vi "CC命令发送.vi"(8 "error in (no error)":errorcluster caption="错误输入（无错误）", 11 "MainPage 输入":refnum<class "MainPage.lvclass">) -> (0 "error out":errorcluster caption="错误输出", 3 "MainPage 输出":refnum<class "MainPage.lvclass">)   [LabVIEW 2019, in "MainPage.lvlib" / "MainPage.lvclass"]
uses:
  MainPage.lvclass
  MainPage.lvclass/MainPage.ctl
panel:
  # "简略版本，后续修改"
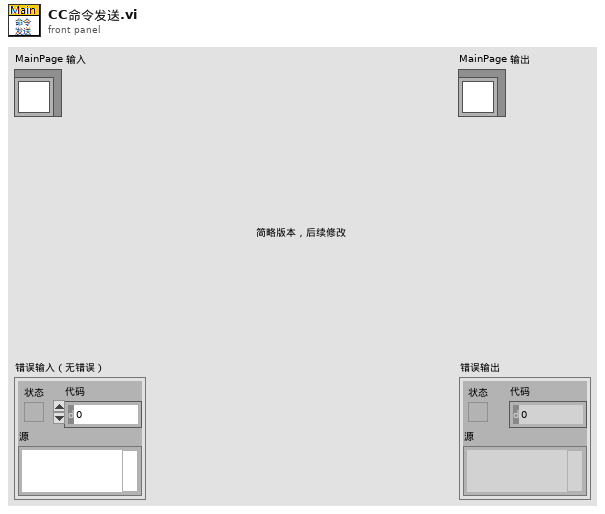
[diagram p1: front panel]
types:
  T1 = typedef "MainPage.lvlib/MainPage.lvclass/DataRef_通讯接口.ctl" = cluster{"连接方式":enum16{"网口(客服端)", "网口(服务端)", "串口"}, "VISA串口名称":refnum<visa-resource-name>, "服务端识别":cluster{"本机IP":string, "本机端口":u16, "当前目标":string, "服务端侦听ID":refnum<k5>}, "客服端识别":cluster{"客P-主IP:Port":string}, "客服端记录":map{string, refnum<k5>}, "服务端接口记录":map{string, refnum<k5>}}
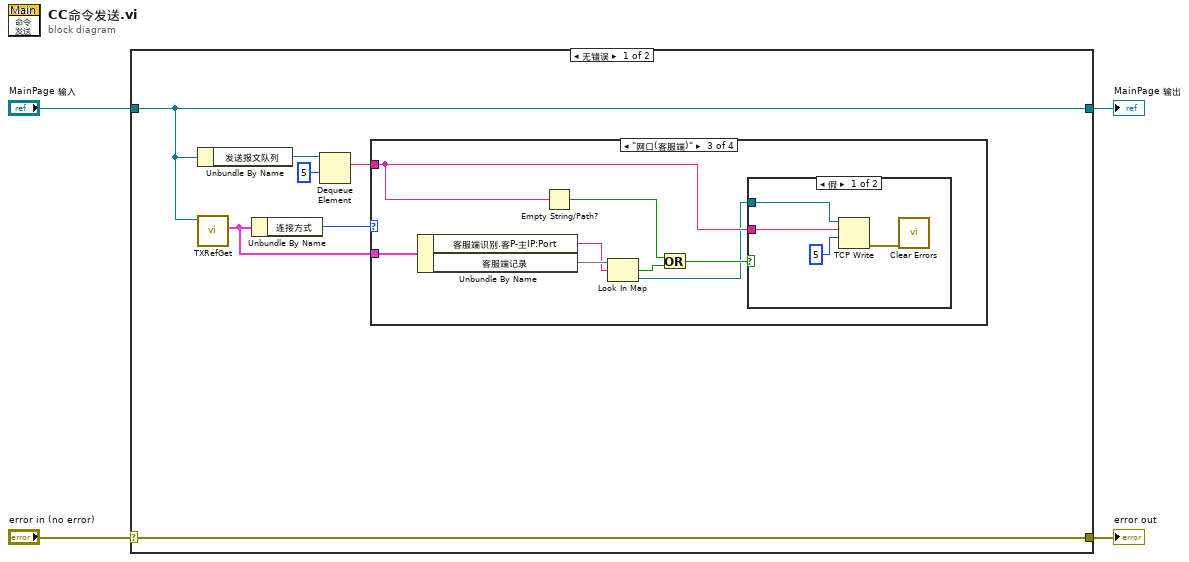
[diagram p0: block diagram]
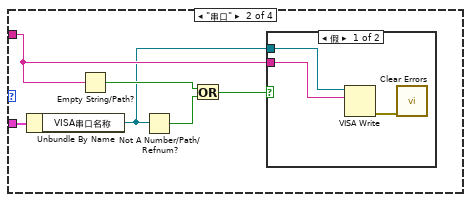
[diagram p3: hidden frame]
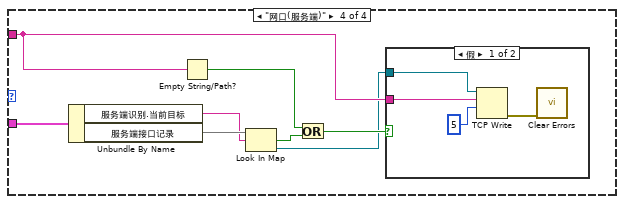
[diagram p6: hidden frame]
diagram:
  n1 = case shown="无错误" "error in (no error)" {
    selector: "error in (no error)" -> [w11 w46]
    tunnel: [w11 w46] -> w3
    tunnel: [w8 w45] -> w1
    tunnel: "MainPage 输入" -> [w8 w45]
    frame No Error {
      n2 = Unbundle By Name(w8) -> ("发送报文队列"=w10:refnum<queue>)
      n3 = call-dynamic "TXRefGet.vi"("MainPage 输入"=w8) -> ("通讯接口数据"=w6:T1)  [unwired: 6 in, 4 out]
      n4 = Unbundle By Name(w6) -> ("连接方式"=w7:enum16{"网口(客服端)", "网口(服务端)", "串口"})
      n5 = Dequeue Element(queue=w10, timeout in ms (-1)=5 ("超时毫秒(-1)")) -> (element=w5:string)  [unwired: 1 in, 3 out]
      n6 = case shown="\"网口(客服端)\"" w7 {
        tunnel: w6 -> [_ w17 w26 w38]
        tunnel: w5 -> [_ w13 w22 w34]
        frame Default {
        }
        frame "串口" {
          n7 = Unbundle By Name(w17) -> ("VISA串口名称"=w12:refnum<visa-resource-name>)
          n8 = Empty String/Path?(string/path=w13) -> (empty?=w15:bool)
          n9 = Not A Number/Path/Refnum?(number/path/refnum=w12) -> (NaN/Path/Refnum?=w16:bool)
          n10 = Or(x=w15, y=w16) -> (x .or. y?=w14:bool)
          n11 = case shown="假" w14 {
            tunnel: w13 -> [w19 _]
            tunnel: w12 -> [w20 _]
            frame False {
              n12 = VISA Write(VISA resource name=w20, write buffer=w19) -> (error out=w18:errorcluster)  [unwired: 1 in, 2 out]
              n13 = call <vilib>:"Clear Errors.vi"("error in (no error)"=w18) -> ()  [unwired: 5 in, 2 out]
            }
            frame True {
            }
          }
        }
        frame "网口(客服端)" {
          n14 = Unbundle By Name(w26) -> ("客服端识别.客P-主IP:Port"=w27:string, "客服端记录"=w28:map{string, refnum<k5>})
          n15 = Empty String/Path?(string/path=w22) -> (empty?=w25:bool)
          n16 = Look In Map(map=w28, key=w27) -> (key not found?=w24:bool, value=w21:refnum<k5>)  [unwired: 1 in]
          n17 = Or(x=w25, y=w24) -> (x .or. y?=w23:bool)
          n18 = case shown="假" w23 {
            tunnel: w22 -> [w31 _]
            tunnel: w21 -> [w32 _]
            frame False {
              n19 = TCP Write(connection ID=w32, data in=w31, 9:5 ("超时毫秒(25000)")) -> (error out=w29:errorcluster)  [unwired: 1 in, 2 out]
              n20 = call <vilib>:"Clear Errors.vi"("error in (no error)"=w29) -> ()  [unwired: 5 in, 2 out]
            }
            frame True {
            }
          }
        }
        frame "网口(服务端)" {
          n21 = Unbundle By Name(w38) -> ("服务端识别.当前目标"=w39:string, "服务端接口记录"=w40:map{string, refnum<k5>})
          n22 = Empty String/Path?(string/path=w34) -> (empty?=w37:bool)
          n23 = Look In Map(map=w40, key=w39) -> (key not found?=w36:bool, value=w33:refnum<k5>)  [unwired: 1 in]
          n24 = Or(x=w37, y=w36) -> (x .or. y?=w35:bool)
          n25 = case shown="假" w35 {
            tunnel: w34 -> [w43 _]
            tunnel: w33 -> [w44 _]
            frame False {
              n26 = TCP Write(connection ID=w44, data in=w43, 9:5 ("超时毫秒(25000)")) -> (error out=w41:errorcluster)  [unwired: 1 in, 2 out]
              n27 = call <vilib>:"Clear Errors.vi"("error in (no error)"=w41) -> ()  [unwired: 5 in, 2 out]
            }
            frame True {
            }
          }
        }
      }
    }
    frame Error {
    }
  }
  "error out" <- w3
  "MainPage 输出" <- w1
